vi "userpassReceptor.vi"(4 "error in (no error)":errorcluster, 7 "connection ID":refnum<k5>) -> (0 "error out":errorcluster, 1 "password":string, 2 "user":string, 3 "connection ID out":refnum<k5>)   [LabVIEW 2010]
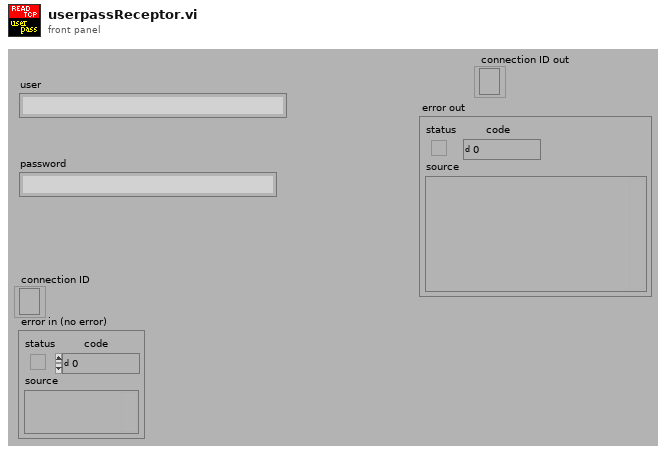
[diagram p1: front panel]
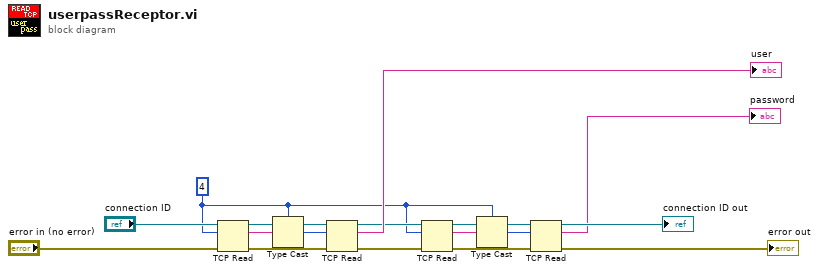
[diagram p0: block diagram]
diagram:
  w2 = 4 ("bytes to read")
  n1 = TCP Read(connection ID="connection ID", bytes to read=w2, error in (no error)="error in (no error)") -> (connection ID out=w17:refnum<k5>, data out=w13:string, error out=w16:errorcluster)  [unwired: 2 out]
  n2 = Type Cast(type=w2, x=w13) -> (*(type *) &x=w12:i32)
  n3 = TCP Read(connection ID=w17, bytes to read=w12, error in (no error)=w16) -> (connection ID out=w6:refnum<k5>, data out=→"user":string, error out=w5:errorcluster)  [unwired: 2 out]
  n4 = TCP Read(connection ID=w6, bytes to read=w2, error in (no error)=w5) -> (connection ID out=w10:refnum<k5>, data out=w8:string, error out=w9:errorcluster)  [unwired: 2 out]
  n5 = Type Cast(type=w2, x=w8) -> (*(type *) &x=w7:i32)
  n6 = TCP Read(connection ID=w10, bytes to read=w7, error in (no error)=w9) -> (connection ID out=→"connection ID out":refnum<k5>, data out=→"password":string, error out=→"error out":errorcluster)  [unwired: 2 out]
